vi "subTiE_SetCubeBottom.vi"(6 "Ref":T2 caption="Ref (can be hidden)", 7 "TI-Ctrl":T1={"Obj"=5, "Cube Bottom"=1, "Cube Top"=6, "PFS-Ctrl"={"PFS IO"=FALSE, "PSF Err"=FALSE, "PSF Pos"=0}, "Z-Ctrl"={"Z-pos"=499.225, "Home"=FALSE, "Sensitivity"=1}, "Condenser"=2, "Lightpath"=enum."EYE"} {"Condenser" items=["A"=1, "DICN2"=2, "- empty 3 -"=3, "- empty 4 -"=4, "- empty 5 -"=5, "- empty 6 -"=6]; "Z-Ctrl"."Sensitivity" min=1 max=3 step=1 scale=1.0..3.0; "PFS-Ctrl"."PSF Pos" scale=0.0..16400.0; "Cube Top" items=["Cy5"=1, "RFP"=2, "DM532"=3, "DM488"=4, "DM405"=5, "- empty 6 -"=6]; "Cube Bottom" items=["- empty 1 -"=1, "- empty 2 -"=2, "EM585/65"=3, "EM525/50"=4, "EM460/50"=5, "DIC"=6]; "Obj" items=["20x/.75 Dry PFS"=1, "40x/1.3 Oil PFS"=2, "60x/1.4 Oil PFS"=3, "- empty 4 -"=4, "- empty 5 -"=5, "- empty 6 -"=6]}) -> ()   [LabVIEW 2015]
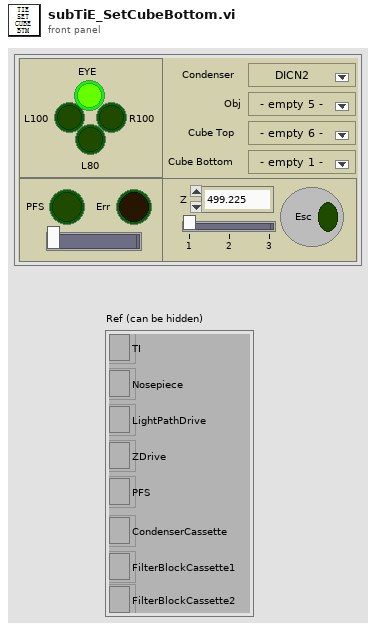
[diagram p1: front panel]
types:
  T1 = cluster{"Obj":u16, "Cube Bottom":u16, "Cube Top":u16, "PFS-Ctrl":cluster{"PFS IO":bool, "PSF Err":bool, "PSF Pos":u32}, "Z-Ctrl":cluster{"Z-pos":dbl, "Home":bool, "Sensitivity":u8}, "Condenser":u16, "Lightpath":enum32{"EYE", "L100", "R100", "L80"}}
  T2 = cluster{"TI":refnum<k7>, "Nosepiece":refnum<k7>, "LightPathDrive":refnum<k7>, "ZDrive":refnum<k7>, "PFS":refnum<k7>, "CondenserCassette":refnum<k7>, "FilterBlockCassette1":refnum<k7>, "FilterBlockCassette2":refnum<k7>}
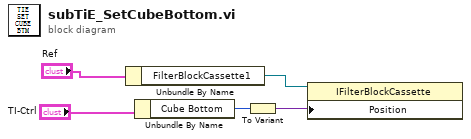
[diagram p0: block diagram]
diagram:
  n1 = Unbundle By Name("Ref") -> ("FilterBlockCassette1"=w5:refnum<k7>)
  n2 = Unbundle By Name("TI-Ctrl") -> ("Cube Bottom"=w1:u16)
  n3 = To Variant(anything=w1) -> (Variant=w4:variant)
  n4 = property class="IFilterBlockCassette"(reference=w5, "Position"=w4) -> ()  [unwired: 1 in, 2 out]
